vi "Create Transaction List.vi"(1 "Source Types":cluster{"Types":T1[]}[](array[cluster]), 2 "Hold":T4, 3 "Volts":bool, 4 "Sources":T3[](array[typedef])) -> (0 "Transactions":T2[](array[typedef]))   [LabVIEW 2009]
uses:
  Apps/Yes No Button.ctl
  Dataset Source.ctl
  Dataset Transaction Id.ctl
  Dataset Type.ctl
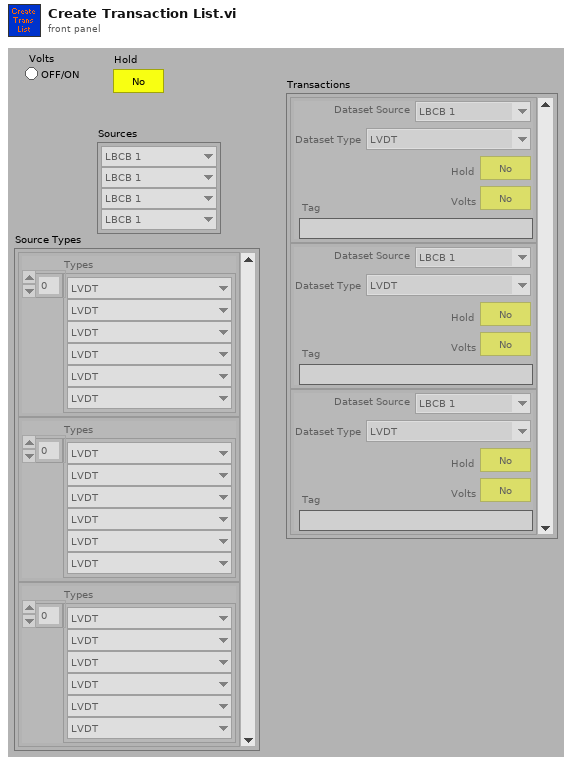
[diagram p1: front panel]
types:
  T1 = typedef "Dataset Type.ctl" = enum16{"LVDT", "Load Cell", "Actuator Command", "Servo Error", "Displacement Command", "Displacement", "Force"}
  T2 = typedef "Dataset Transaction Id.ctl" = cluster{"Dataset Source":T3, "Dataset Type":T1, "Hold":T4, "Volts":T4, "Tag":string}
  T3 = typedef "Dataset Source.ctl" = enum16{"LBCB 1", "LBCB 2", "Combined", "External Sensors"}
  T4 = typedef "Yes No Button.ctl" = bool
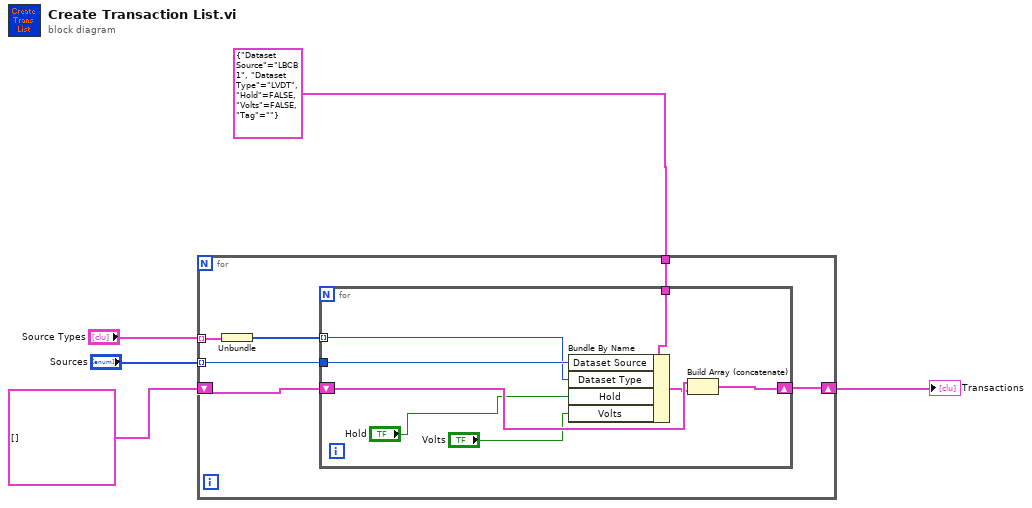
[diagram p0: block diagram]
diagram:
  n1 = for {
    tunnel: T2 {"Dataset Source"=enum."LBCB 1", "Dataset Type"=enum."LVDT", "Hold"=FALSE, "Volts"=FALSE, "Tag"=""} ("Dataset Trans Id") -> [w11]
    shift-right: [w8] -> w3
    shift-left: T2[] [] -> [w9]
    tunnel: "Sources" -> [w10] mode=indexing
    tunnel: "Source Types" -> [w7] mode=indexing
    n2 = Unbundle(w7) -> ("Types"=w6:T1[])
    n3 = for {
      tunnel: w11 -> [w19]
      shift-right: [w18] -> w8
      shift-left: w9 -> [w17]
      tunnel: w10 -> [w16]
      tunnel: w6 -> [w14] mode=indexing
      n4 = Bundle By Name(cluster=w19, "Dataset Source"=w16, "Dataset Type"=w14, "Hold"="Hold", "Volts"="Volts") -> (w15:T2)
      n5 = Build Array (concatenate)(w17, w15) -> (w18:T2[])
    }
  }
  "Transactions" <- w3
